vi "GetNumberOfHammers.vi"(2 "config":T1[](array[typedef])) -> (7 "hammers":i16, 9 "hammerIndex":i32)   [LabVIEW 2017]
uses:
  MainFGV/Settings/config_board.ctl
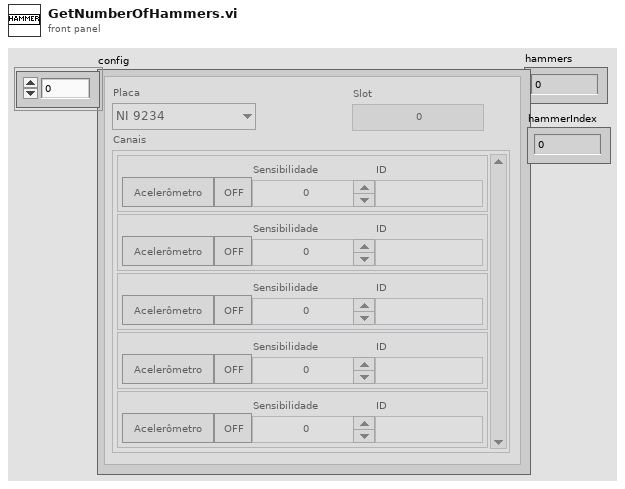
[diagram p1: front panel]
types:
  T1 = typedef "config_board.ctl" = cluster{"board":enum16{"NI 9234", "NI 9205", "Não aplicável"}, "channels":cluster{"type":bool, "active":bool, "sens":dbl, "ID":string}[], "Slot":i32}
  T2 = cluster{"type":bool, "active":bool, "sens":dbl, "ID":string}[]
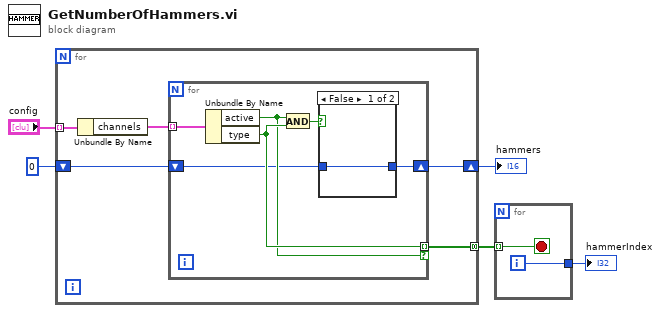
[diagram p0: block diagram]
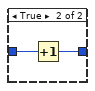
[diagram p2: hidden frame]
diagram:
  n1 = for {
    tunnel: "config" -> [w10] mode=indexing
    tunnel: [w8] -> w3 mode=concatenating
    shift-right: [w6] -> w1
    shift-left: i16 0 -> [w7]
    n2 = Unbundle By Name(w10) -> ("channels"=w9:T2)
    n3 = for {
      tunnel: w9 -> [w16] mode=indexing
      tunnel: [w15] -> w8 mode=indexing if=w14
      shift-right: [w11] -> w6
      shift-left: w7 -> [w12]
      n4 = Unbundle By Name(w16) -> ("active"=w14:bool, "type"=w15:bool)
      n5 = And(x=w14, y=w15) -> (x .and. y?=w13:bool)
      n6 = case shown="False" w13 {
        tunnel: w12 -> [w17 w19]
        tunnel: [w17 w18] -> w11
        frame False {
        }
        frame True {
          n7 = Increment(x=w19) -> (x+1=w18:i16)
        }
      }
    }
  }
  "hammers" <- w1
  n8 = for {
    tunnel: [w21] -> w4
    tunnel: w3 -> [w20] mode=indexing
    i -> [w21]
    stop <- w20 stop-if-true
  }
  "hammerIndex" <- w4
